vi "$打开CSV保存路径.vi"   [LabVIEW 2017]
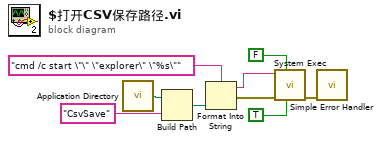
[diagram p0: block diagram]
diagram:
  n1 = call <vilib>:"Application Directory.vi"() -> ("Application Directory"=w5:path)
  n2 = Build Path(base path=w5, name or relative path="CsvSave") -> (appended path=w3:path)
  n3 = Format Into String(format string="cmd /c start \"\" \"explorer\" \"%s\"", w3) -> (resulting string=w8:string, error out=w9:errorcluster)  [unwired: 2 in]
  n4 = call <vilib>:"System Exec.vi"("run minimized? (F)"=TRUE, "wait until completion? (T)"=FALSE, "error in (no error)"=w9, "command line"=w8) -> ("error out"=w2:errorcluster)  [unwired: 4 in, 3 out]
  n5 = call <vilib>:"Simple Error Handler.vi"("error in (no error)"=w2) -> ()  [unwired: 4 in, 5 out]
